vi "Notify Launcher.vi"(8 "error in (no error)":errorcluster, 10 "Notification":string, 11 "Measure Controller in":refnum<class "Process Controller.lvclass">) -> (0 "error out":errorcluster, 3 "Measure Controller out":refnum<class "Process Controller.lvclass">)   [LabVIEW 2016, in "Process Controller.lvclass"]
uses:
  Process Controller.lvclass
  Process Controller.lvclass/Process Controller.ctl
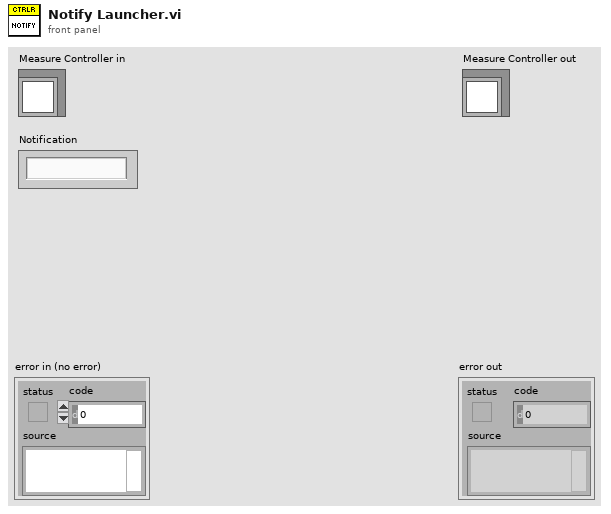
[diagram p1: front panel]
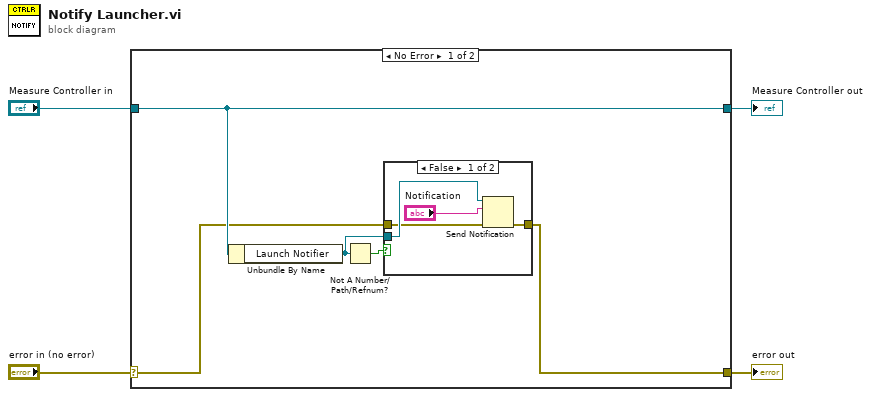
[diagram p0: block diagram]
diagram:
  n1 = case shown="No Error" "error in (no error)" {
    selector: "error in (no error)" -> [w6 w16]
    tunnel: [w5 w16] -> w3
    tunnel: [w7 w15] -> w1
    tunnel: "Measure Controller in" -> [w7 w15]
    frame No Error {
      n2 = Unbundle By Name(w7) -> ("Launch Notifier"=w9:refnum<notifier>)
      n3 = Not A Number/Path/Refnum?(number/path/refnum=w9) -> (NaN/Path/Refnum?=w8:bool)
      n4 = case shown="False" w8 {
        tunnel: w9 -> [w12 _]
        tunnel: w6 -> [w11 w14]
        tunnel: [w10 w14] -> w5
        frame False {
          n5 = Send Notification(notification="Notification", notifier=w12, error in (no error)=w11) -> (error out=w10:errorcluster)  [unwired: 1 out]
        }
        frame True {
        }
      }
    }
    frame Error {
    }
  }
  "error out" <- w3
  "Measure Controller out" <- w1
